vi "deltaHRT.vi"(9 "data input":T2, 10 "setpoints":T1={"target clarified turbidity (NTU)"=0.3, "flocculator volume (L)"=0.0, "clarifier volume (L)"=0.0, "dose updates per HRT"=1} {"target clarified turbidity (NTU)" min=0.1 max=5.0 step=0.01; "dose updates per HRT" min=1 max=1000 step=1}, 11 "seconds since 1Jan1904":timestamp) -> (1 "new interval":bool, 2 "sum HRT":dbl, 3 "delta HRT":dbl)   [LabVIEW 2014]
uses:
  setpoints.ctl
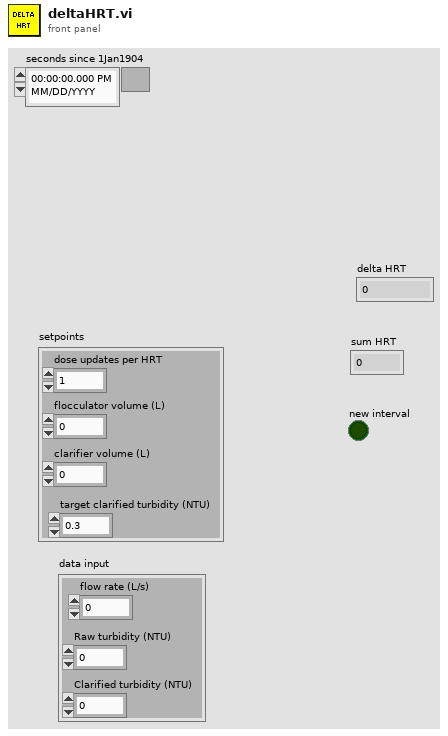
[diagram p1: front panel]
types:
  T1 = typedef "setpoints.ctl" = cluster{"target clarified turbidity (NTU)":dbl, "flocculator volume (L)":dbl, "clarifier volume (L)":dbl, "dose updates per HRT":u32}
  T2 = cluster{"Clarified turbidity (NTU)":dbl, "Raw turbidity (NTU)":dbl, "flow rate (L/s)":dbl}
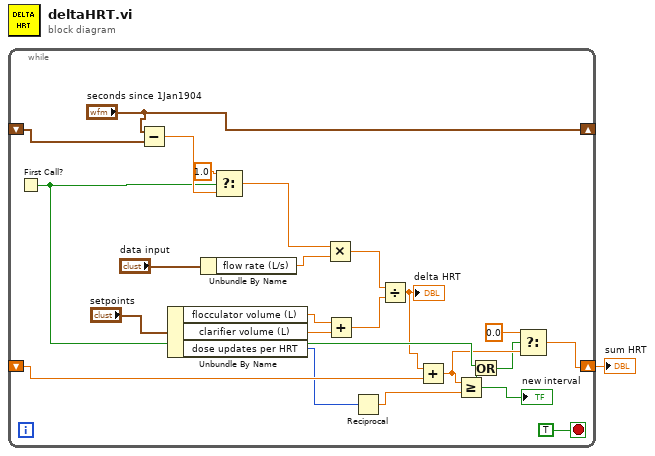
[diagram p0: block diagram]
diagram:
  n1 = while {
    shift-right: ["seconds since 1Jan1904"] -> _
    shift-left: _ -> [w16]
    shift-right: [w9] -> w1
    shift-left: _ -> [w10]
    stop <- TRUE stop-if-true
    n2 = First Call?() -> (First Call?: T/F=w8:bool)
    n3 = Subtract(x="seconds since 1Jan1904", y=w16) -> (x-y=w14:dbl)
    n4 = Unbundle By Name("setpoints") -> ("flocculator volume (L)"=w21:dbl, "clarifier volume (L)"=w20:dbl, "dose updates per HRT"=w3:u32)
    n5 = Unbundle By Name("data input") -> ("flow rate (L/s)"=w22:dbl)
    n6 = Select(t=1.0, s=w8, f=w14) -> (s? t:f=w12:dbl)
    n7 = Multiply(x=w12, y=w22) -> (x*y=w19:dbl)
    n8 = Add(x=w21, y=w20) -> (x+y=w18:dbl)
    n9 = Reciprocal(x=w3) -> (1/x=w2:dbl)
    n10 = Divide(x=w19, y=w18) -> (x/y=w6:dbl)
    "delta HRT" <- w6
    n11 = Add(x=w6, y=w10) -> (x+y=w5:dbl)
    n12 = Greater Or Equal?(x=w5, y=w2) -> (x >= y?=w7:bool)
    "new interval" <- w7
    n13 = Or(x=w8, y=w7) -> (x .or. y?=w4:bool)
    n14 = Select(t=0.0, s=w4, f=w5) -> (s? t:f=w9:dbl)
  }
  "sum HRT" <- w1
